vi "cumplimiento.vi"(8 "error in (no error)":errorcluster, 9 "mediciones in":T1, 10 "Tabla in":string[][](array[string])) -> (0 "error out":errorcluster, 1 "mediciones out":T1, 2 "Tabla out":string[][](array[string]), 3 "Prueba04 out":refnum<class "Prueba04.lvclass">)   [LabVIEW 2019, in "Prueba04.lvclass"]
uses:
  Prueba04.lvclass
panel:
  out "cumpimiento":string
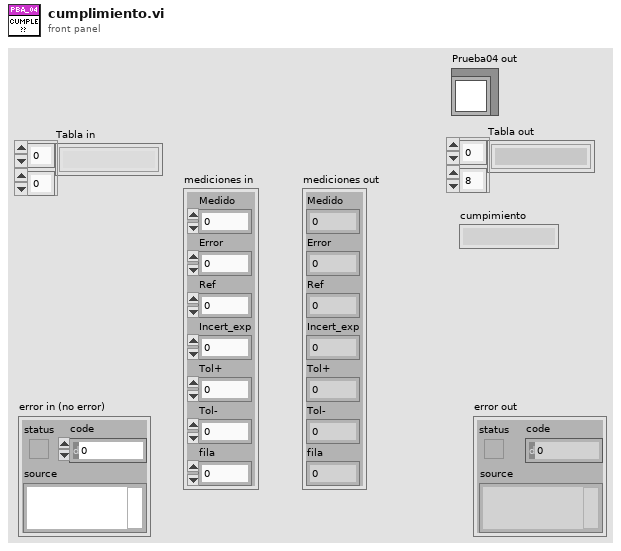
[diagram p1: front panel]
types:
  T1 = cluster{"Medido":dbl, "Error":dbl, "Ref":dbl, "Incert_exp":dbl, "Tol+":dbl, "Tol-":dbl, "fila":i32}
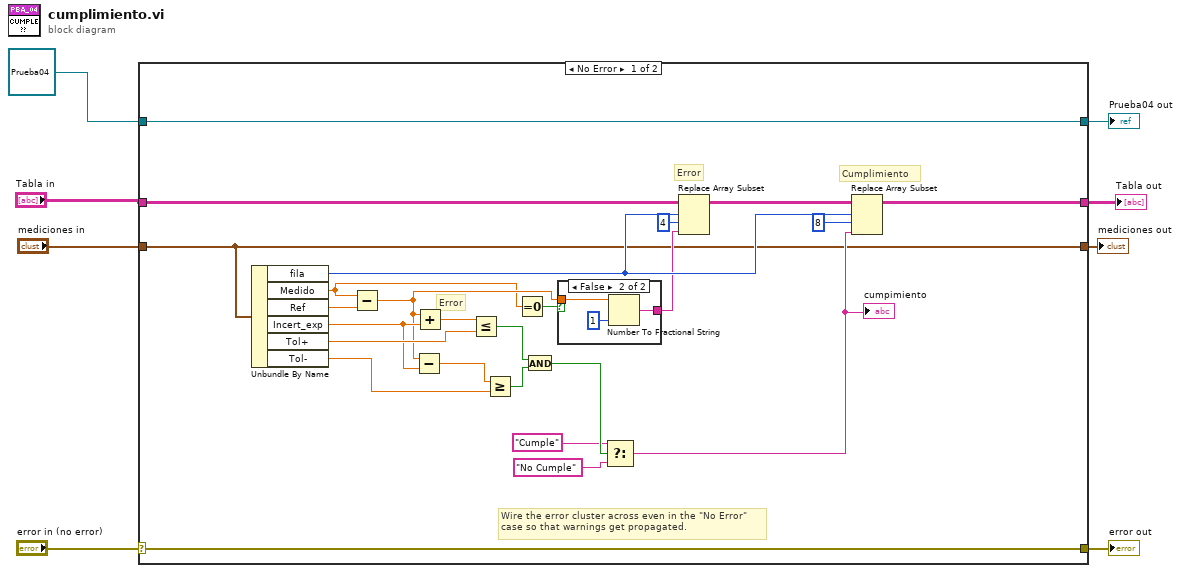
[diagram p0: block diagram]
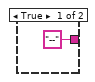
[diagram p2: hidden frame]
diagram:
  n1 = case shown="No Error" "error in (no error)" {
    selector: "error in (no error)" -> [w32 w41]
    tunnel: [w32 w41] -> w7
    tunnel: [w33 w40] -> w5
    tunnel: refnum<class "Prueba04.lvclass"> refnum ("Prueba04 in") -> [w33 w40]
    tunnel: "Tabla in" -> [w11 w39]
    tunnel: "mediciones in" -> [w10 w38]
    tunnel: [w10 w38] -> w1
    tunnel: [w9 w39] -> w3
    frame No Error {
      # "Cumplimiento"
      # "Error"
      # "Error"
      # "Wire the error cluster across even in the \"No Error\"\ncase so that warnings get propagated."
      n2 = Unbundle By Name(w10) -> ("fila"=w17:i32, "Medido"=w12:dbl, "Ref"=w24:dbl, "Incert_exp"=w22:dbl, "Tol+"=w23:dbl, "Tol-"=w21:dbl)
      n3 = Subtract(x=w12, y=w24) -> (x-y=w13:dbl)
      n4 = Subtract(x=w13, y=w22) -> (x-y=w28:dbl)
      n5 = Add(x=w13, y=w22) -> (x+y=w31:dbl)
      n6 = Less Or Equal?(x=w31, y=w23) -> (x <= y?=w30:bool)
      n7 = Greater Or Equal?(x=w28, y=w21) -> (x >= y?=w29:bool)
      n8 = Equal To 0?(x=w12) -> (x = 0?=w14:bool)
      n9 = And(x=w30, y=w29) -> (x .and. y?=w27:bool)
      n10 = case shown="False" w14 {
        tunnel: w13 -> [_ w37]
        tunnel: ["--" w35] -> w15
        frame True {
        }
        frame False {
          n11 = Number To Fractional String(number=w37, precision (6)=i16 1) -> (F-format string=w35:string)  [unwired: 2 in]
        }
      }
      n12 = Select(t="Cumple", s=w27, f="No Cumple") -> (s? t:f=w20:string)
      "cumpimiento" <- w20
      n13 = Replace Array Subset(array=w11, new element=w15, index (row)=w17, index (col)=4 ("disabled index (col)")) -> (w18:string[][])
      n14 = Replace Array Subset(array=w18, new element=w20, index (row)=w17, index (col)=8 ("index (row)")) -> (w9:string[][])
    }
    frame Error {
    }
  }
  "error out" <- w7
  "Prueba04 out" <- w5
  "Tabla out" <- w3
  "mediciones out" <- w1
